vi "Ver 1.8.vi"() -> ()   [LabVIEW 2015]
uses:
  <instrlib>/Keithley 622x LV 2009/Configure/Source/Typedefs/KE622x -- Current Range.ctl
  <instrlib>/Keithley 622x LV 2009/Configure/Source/Typedefs/KE622x -- Current Ranges.ctl
  <instrlib>/Keithley 622x LV 2009/Typedefs/KE622x -- On Off Control.ctl
  <instrlib>/Keithley 622x LV 2009/Configure/Source/Typedefs/KE622x -- Voltage Limit.ctl
  <instrlib>/Keithley 622x LV 2009/Utility/Typedefs/KE622x -- Instrument Type.ctl
  <instrlib>/Keithley 2000/Public/Configure/Configure DC Volts.vi
  <userlib>/LV-Link3/PolySubVIs/DtCreateAinChan.vi
  <userlib>/LV-Link3/PolySubVIs/DtOLReadSingle.vi
  <instrlib>/Keithley 2000/Keithley 2000.lvlib
  <instrlib>/Keithley 622x LV 2009/Keithley 622x.lvlib
panel:
  out "MULTIPLE GRAPHS":cluster{dbl[], dbl[]}[](graph)
  in  "X-Axis":T1(ring)
  in  "Range":u8(ring)=20 items=["100nV", "200nV", "500nV", "1µV", "2µV", "5µV", "10µV", "20µV", "50µV", "100µV", "200µV", "500µV", "1mV", "2mV", "5mV", "10mV", "20mV", "50mV", "100mV", "200mV", "500mV", "1V"]
  in  "Display Type copy":u16(ring) items=["X %", "Y %", "X Calibrated", "Y Calibrated", "Mag %", "Mag Calibrated", "Phase Degrees", "Ratio", "ADC 1", "ADC 2", "ADC 3", "ADC 4 ", "Noise %", "Noise Calibrated", "Ref Frequency", "", ""]
  out "Units copy":string
  out "Display copy":dbl format="%.3f"
  out "Overload":bool
  out "Display":dbl format="%.3f"
  out "Units":string
  in  "Display Type":u16(ring) items=["X %", "Y %", "X Calibrated", "Y Calibrated", "Mag %", "Mag Calibrated", "Phase Degrees", "Ratio", "ADC 1", "ADC 2", "ADC 3", "ADC 4 ", "Noise %", "Noise Calibrated", "Ref Frequency", "", ""]
  in  "Time Constant":u16(ring) items=["MIN", "1ms", "3ms", "10ms", "30ms", "100ms", "300ms", "1s", "3s", "10s", "30s", "100s", "300s"]
  in  "Slope":u8(ring) items=["6db/octave", "12dB/octave"]
  in  "Dynamic Reserve":u16(ring) items=["High Stability", "Normal", "High Reserve"]
  in  "Auto Sensitivity":bool
  in  "Auto Measure":bool
  out "Task out":i32
  out "daq_error out":errorcluster
  out "6221_error_out":errorcluster
  out "2000_error_out":errorcluster
  out "5110_error_out":errorcluster
  out "Input Mode":i32(ring) items=[" Voltage Input (A or A-B) ", "Current Input 10E6 V/A", "Current Input 10E8 V/A"]
  out "5110":refnum<visa-resource-name>
  in  "GPIB Address":i8=12 min=1 max=32 step=1
  out "DAQ":dbl format="%#_13g"
  out "2000":dbl format="%#_13g"
  in  "Device":string(combo)
  in  "Channels":string="0"
  in  "Number \nof points":i32
  in  "Folder\nprename":string
  out "TIME GRAPH":cluster{dbl[], dbl[]}[](graph)
  out "T0":u32
  out "LIMIT":bool
  out "LIMIT":bool
  out "Error Code":string
  in  "Comments":string
  out "file":refnum<file>
  out "2000":refnum<visa-resource-name>
  out "6221":refnum<visa-resource-name>
  out "Step  (A)":dbl=5e-05 format="%#_3p"
  in  "Stop\ncurrent (A)":dbl=0.002 format="%#_6p"
  in  "Start \ncurrent (A)":dbl=0.001 format="%#_6p"
  in  "Check For SCPI Errors? (T)":bool=TRUE
  out "Interlock Tripped?":bool
  out "Compliance?":bool
  in  "Turn Off Output \nIf Compliance?":bool=TRUE
  in  "Turning ON/OFF\ncurrent output":T2=enum."On"
  in  "Range Selection":T3={"Auto Range?"=TRUE, "Man / Selected\nRange"=enum."2nA"}
  # "FILE CONFIGURATION"
  # "ADMIN PANEL"
  # "KEITHLEY 6221 CONFIGURATION (ADMIN ONLY)"
  # "KEITHLEY DAQ CONFIGURATION (ADMIN ONLY)"
  # "READINGS"
  # "PRINCETON LOCK-IN AMP (ADMIN ONLY)"
  # "I don't know what the hell it is,\njust don't touch it"
  # "SENSITIVITY"
  # "INPUT CONFIGURATION"
  # "START, STOP, STEP, CONFIGURATION"
  # "IF ON"
  # "Output Channels Time - Constant \nSlope & Dynamic Reserve"
  # "Compliance = Limiting output voltage\nThis switch determines if we want to switch \noff the current output if wee exceed compliance"
  # "LOCK-IN READINGS"
  # "RIGHT DISPLAY"
  # "LEFT DISPLAY"
  # "There is a safe switch at \nthe back of the instrument \nThis indicator shows if it is on"
  # "You have hit a damn jackpot \nby exceeding the limited voltage\nCongrats"
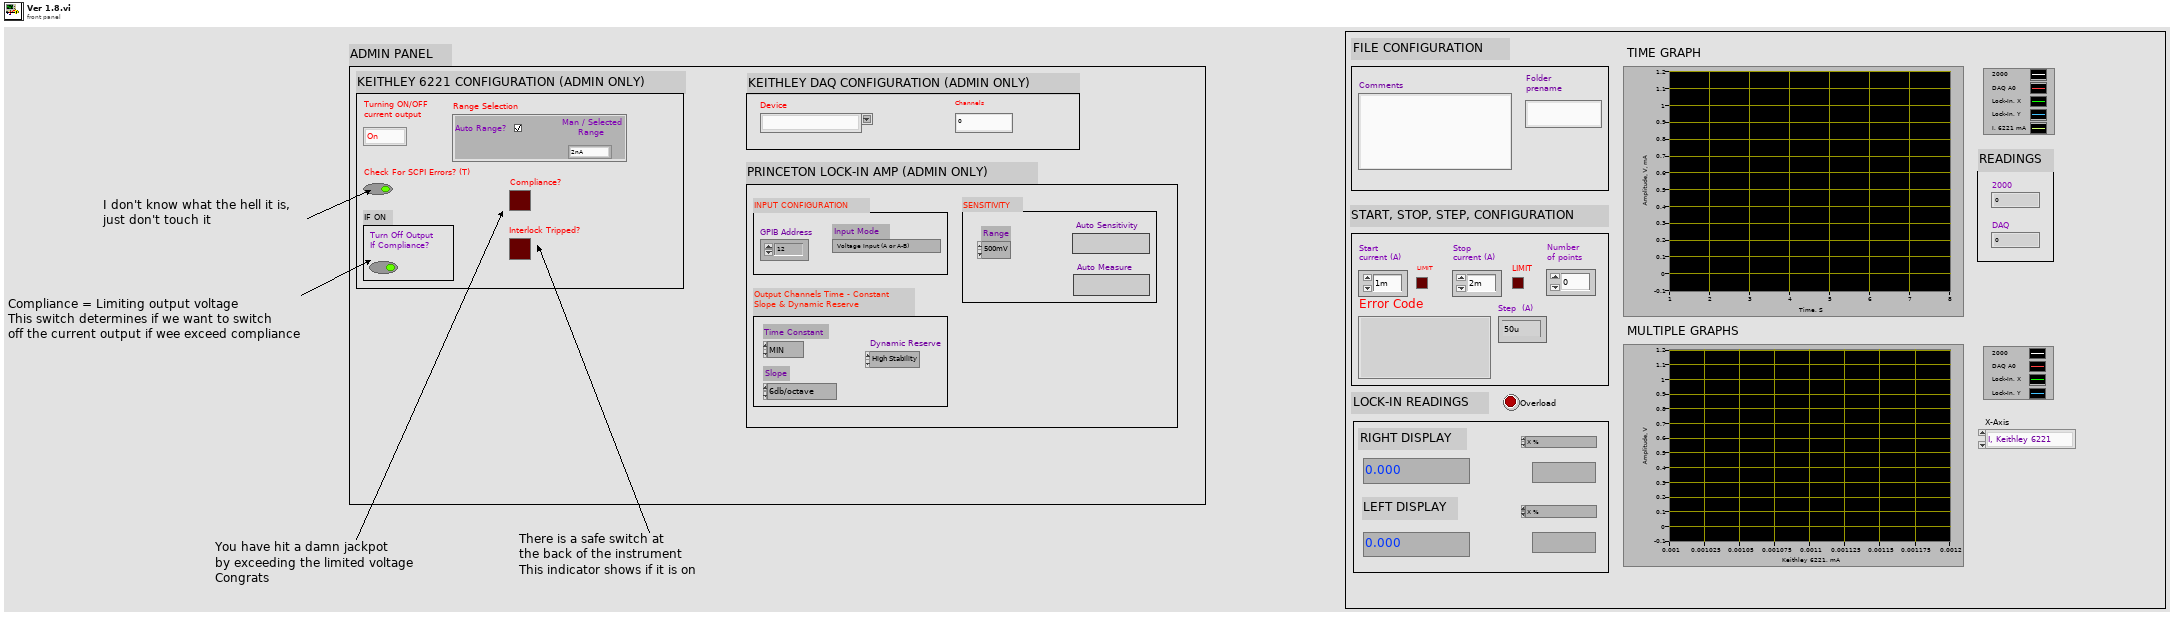
[diagram p1: front panel]
types:
  T1 = enum16{"I, Keithley 6221", "V, Keithley 2000", "V, Keithley DAQ", "V, Lock-In X", "V, Lock-In Y"}
  T2 = typedef "Keithley 622x.lvlib/KE622x -- On Off Control.ctl" = enum16{"Off", "On"}
  T3 = typedef "Keithley 622x.lvlib/KE622x -- Current Range.ctl" = cluster{"Auto Range?":bool, "Man / Selected\nRange":T4}
  T4 = typedef "Keithley 622x.lvlib/KE622x -- Current Ranges.ctl" = enum16{"2nA", "20nA", "200nA", "2uA", "20uA", "200uA", "2mA", "20mA", "100mA"}
  T5 = typedef "Keithley 622x.lvlib/KE622x -- Voltage Limit.ctl" = dbl
  T6 = typedef "Keithley 622x.lvlib/KE622x -- Instrument Type.ctl" = enum16{"KE6220", "KE6221"}
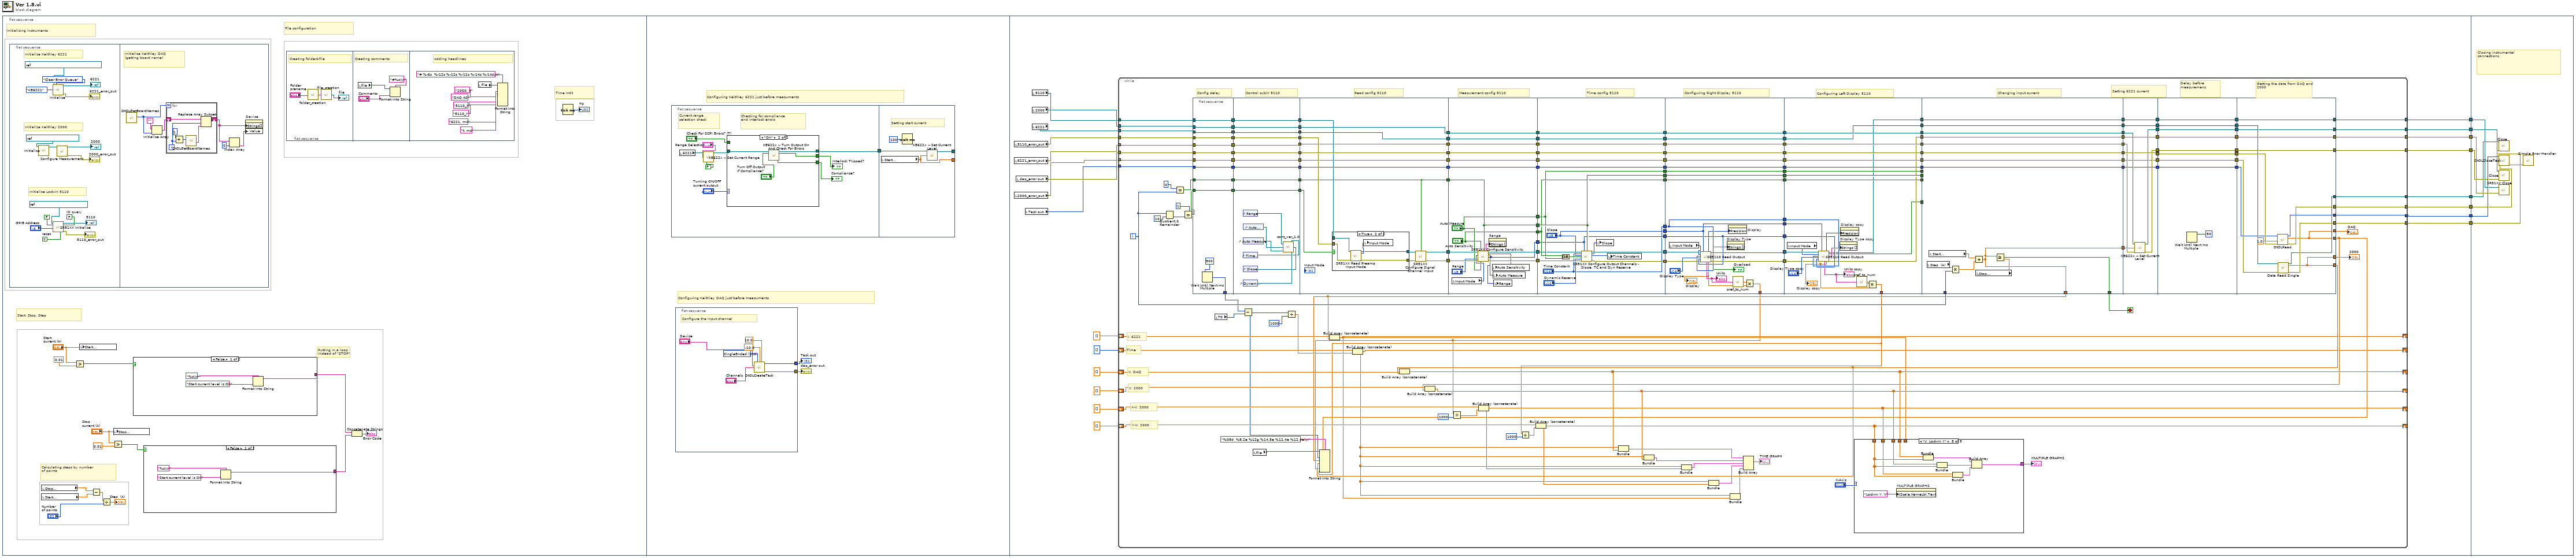
[diagram p0: block diagram]
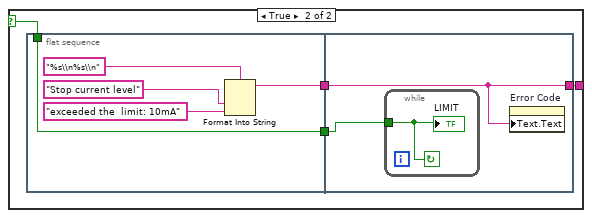
[diagram p2: hidden frame]
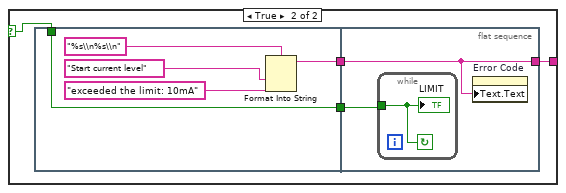
[diagram p3: hidden frame]
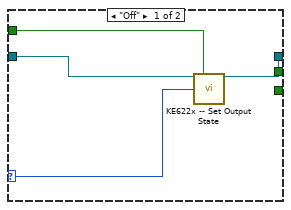
[diagram p4: hidden frame]
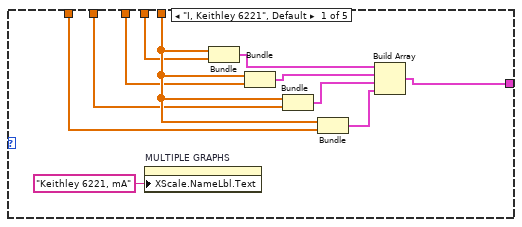
[diagram p5: hidden frame]
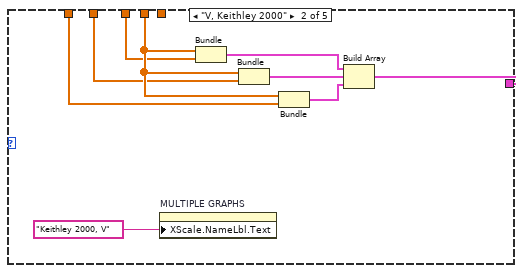
[diagram p6: hidden frame]
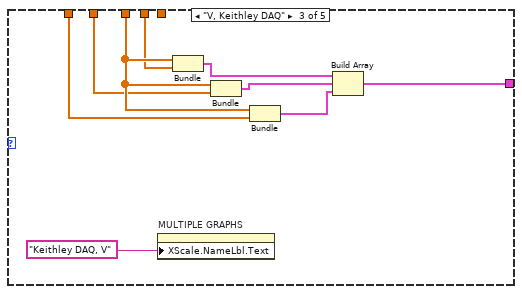
[diagram p7: hidden frame]
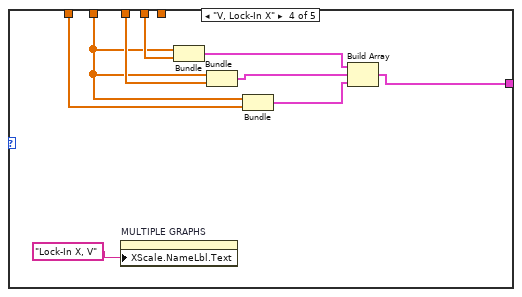
[diagram p8: hidden frame]
diagram:
  n1 = flat-sequence {
    tunnel: [w147] -> w8
    tunnel: [w145] -> w7
    tunnel: [w144] -> w6
    tunnel: [w143] -> w5
    tunnel: [w142] -> w4
    tunnel: [w141] -> w3
    tunnel: [w140] -> w2
    tunnel: [w139] -> w1
    tunnel: w8 -> [w560]
    tunnel: w7 -> [w559]
    tunnel: w6 -> [w558]
    tunnel: w5 -> [w557]
    tunnel: w4 -> [w556]
    tunnel: w3 -> [w555]
    tunnel: w2 -> [w554]
    tunnel: w1 -> [w553]
    frame #0 {
      # "Calculating steps by number\nof points"
      # "Time Intit"
      # "Putting in a loop \ninstead of \"STOP\""
      # "Start, Stop, Step"
      # "Initializing instruments"
      # "File configuration"
      n2 = flat-sequence {
        frame #0 {
          w31 = TRUE  # reset
          w30 = FALSE  # ID query
          # "Initialize Lock-In 5110"
          # "Initialize Keithley 2000"
          # "Initialize Keithley 6221"
          n3 = call <instrlib>:"Initialize.vi"("VISA resource name"=refnum<visa-resource-name> "KEITHLEY_MULTIMETER") -> ("VISA resource name out"=w35:refnum<visa-resource-name>)  [unwired: 17 in, 1 out]
          n4 = call <instrlib>:"Initialize.vi"("VISA resource name"=refnum<visa-resource-name> "KEITHLEY_DC_AC_CURRENT_SOURCE", "Error Queue Option"=enum16{"Clear Error Queue", "Error Query"}."Clear Error Queue", "Instrument Type"=KE622x_--_Instrument_Type."KE6221") -> ("VISA resource name out"=→"6221":refnum<visa-resource-name>, "error out"=→"6221_error_out":errorcluster)  [unwired: 11 in]
          n5 = call "SR51XX Initialize"("VISA session (for class)"=refnum<visa-resource-name> "LOCK_IN_5110_PRINCETON", "Interface"=FALSE, "ID query"=w30, "GPIB Address"="GPIB Address", "reset"=w31) -> ("VISA session"=→"5110":refnum<visa-resource-name>, "error out"=→"5110_error_out":errorcluster)  [unwired: 8 in, 1 out]
          n6 = call-poly <instrlib>:"Configure Measurement.vi"("VISA resource name"=w35) -> ("VISA resource name out"=→"2000":refnum<visa-resource-name>, "error out"=→"2000_error_out":errorcluster)  [unwired: 17 in]
        }
        frame #1 {
          # "Initialize Keithley DAQ \n(getting board name)"
          n7 = call <userlib>:"DtOLGetBoardNames.vi"() -> ("Number of boards"=w40:u32)  [unwired: 9 in, 2 out]
          n8 = Initialize Array("", w40) -> (w42:string[])
          n9 = for {
            N: w40 -> [_]
            shift-right: [w48] -> w45
            shift-left: w42 -> [w49]
            i -> [w47]
            n10 = Add(x=1, y=w47) -> (x+y=w51:i32)
            n11 = call <userlib>:"DtOLGetBoardNames.vi"("Select Board"=w51) -> ("Board Name"=w46:string)  [unwired: 8 in, 2 out]
            n12 = Replace Array Subset(array=w49, new element=w46, index=w47) -> (w48:string[])
          }
          n13 = Index Array(array=w45, index=0) -> (element=w44:string)
          n14 = property on="Device" class="CmbBox"("Strings[]"=w45, "Value"=w44) -> ()  [unwired: 2 in, 2 out]
        }
      }
      n15 = local read "Stop\ncurrent (A)"() -> (w12:dbl)
      n16 = local read "Start \ncurrent (A)"() -> (w11:dbl)
      n17 = Greater?(x="Start \ncurrent (A)", y=T5 0.01) -> (0:w19:bool)
      n18 = local write "Start \ncurrent (A)"("Start \ncurrent (A)") -> ()
      n19 = Subtract(x=w12, y=w11) -> (x-y=w9:dbl)
      n20 = Divide(x=w9, y="Number \nof points") -> (x/y=→"Step  (A)":dbl)
      n21 = Greater?(x="Stop\ncurrent (A)", y=T5 0.01) -> (0:w18:bool)
      n22 = local write "Stop\ncurrent (A)"("Stop\ncurrent (A)") -> ()
      n23 = case shown="False" w19 {
        selector: w19 -> [_ w71]
        tunnel: [w67 w73] -> w17
        frame False {
          n24 = Format Into String(format string="%s\\n", "Start current level is OK" ("false string")) -> (resulting string=w67:string)  [unwired: 2 in, 1 out]
        }
        frame True {
          n25 = flat-sequence {
            tunnel: [w75] -> w72
            tunnel: w71 -> [w74]
            tunnel: [w74] -> w70
            tunnel: [w79] -> w73
            tunnel: w72 -> [w79]
            tunnel: w70 -> [w80]
            frame #0 {
              n26 = Format Into String(format string="%s\\n%s\\n", "Start current level" ("String"), "exceeded the limit: 10mA" ("input 2")) -> (resulting string=w75:string)  [unwired: 2 in, 1 out]
            }
            frame #1 {
              n27 = while {
                tunnel: w80 -> [w81]
                stop <- w81 continue-if-true
                "LIMIT" <- w81
              }
              n28 = property on="Error Code" class="Str"("Text.Text"=w79) -> ()  [unwired: 2 in, 2 out]
            }
          }
        }
      }
      n29 = case shown="False" w18 {
        selector: w18 -> [_ w55]
        tunnel: [w52 w58] -> w16
        frame False {
          n30 = Format Into String(format string="%s\\n", "Start current level is OK" ("false string")) -> (resulting string=w52:string)  [unwired: 2 in, 1 out]
        }
        frame True {
          n31 = flat-sequence {
            tunnel: [w60] -> w57
            tunnel: [w59] -> w56
            tunnel: w55 -> [w59]
            tunnel: [w64] -> w58
            tunnel: w57 -> [w64]
            tunnel: w56 -> [w65]
            frame #0 {
              n32 = Format Into String(format string="%s\\n%s\\n", "Stop current level" ("String"), "exceeded the  limit: 10mA" ("input 2")) -> (resulting string=w60:string)  [unwired: 2 in, 1 out]
            }
            frame #1 {
              n33 = while {
                tunnel: w65 -> [w66]
                stop <- w66 continue-if-true
                "LIMIT" <- w66
              }
              n34 = property on="Error Code" class="Str"("Text.Text"=w64) -> ()  [unwired: 2 in, 2 out]
            }
          }
        }
      }
      n35 = flat-sequence {
        frame #0 {
          # "Creating folder&file"
          n36 = call "folder_creation.vi"("Name"="Folder\nprename") -> ("String"=w83:string)
          n37 = call "file_creation.vi"("String"=w83) -> ("refnum out"=→"file":refnum<file>)
        }
        frame #1 {
          # "Creating comments"
          n38 = local read "file"() -> (w85:refnum<file>)
          n39 = Format Into String(format string="#%s\\n", initial string=w85, "Comments") -> ()  [unwired: 1 in, 2 out]
        }
        frame #2 {
          # "Adding headlines"
          n40 = local read "file"() -> (w95:refnum<file>)
          n41 = Format Into String(format string="# %-6s  %-12s %-12s %-12s %-14s %-14s\\n", initial string=w95, "t, ms" ("input 3"), "6221, mA" ("input 3"), "2000, V" ("input 1"), "DAQ A0" ("input 2"), "5110_X" ("input 3"), "5110_Y " ("input 3")) -> ()  [unwired: 1 in, 2 out]
        }
      }
      n42 = Concatenate Strings(w17, w16) -> (→"Error Code":string)
      n43 = Tick Count (ms)() -> (millisecond timer value=→"T0":u32)
    }
    frame #1 {
      # "Configuring Keithley DAQ just before measuments"
      # "Configuring Keithley 6221 just before measuments"
      n44 = flat-sequence {
        tunnel: [w106] -> w98
        tunnel: [w124] -> _
        tunnel: [w126] -> _
        tunnel: w98 -> [w125]
        frame #0 {
          # "Current range \nselection check"
          # "Checking for compliance\nand interlock errors"
          n45 = local read "6221"() -> (w109:refnum<visa-resource-name>)
          n46 = call <instrlib>:"KE622x -- Set Current Range.vi"("Resource In"=w109, "Current Range In"="Range Selection", "Read Back Set Values? (T)"=FALSE) -> ("Resource Out (dupl)"=w114:refnum<visa-resource-name>)  [unwired: 10 in, 2 out]
          n47 = case shown="\"On\"" "Turning ON/OFF\ncurrent output" {
            selector: "Turning ON/OFF\ncurrent output" -> [w118 _]
            tunnel: [_ w122] -> w112
            tunnel: [_ w121] -> w113
            tunnel: "Check For SCPI Errors? (T)" -> [w117 _]
            tunnel: w114 -> [w115 w120]
            tunnel: [w116 w119] -> w106
            frame "Off" {
              n48 = call <instrlib>:"KE622x -- Set Output State.vi"("Resource In"=w115, "Check For SCPI Errors? (T)"=w117, "Output State"=w118) -> ("Resource Out (dupl)"=w116:refnum<visa-resource-name>)  [unwired: 11 in, 1 out]
            }
            frame "On" {
              n49 = call <instrlib>:"KE622x -- Turn Output On And Check For Errors.vi"("Resource In"=w120, "Turn Off Output If Compliance?"="Turn Off Output \nIf Compliance?") -> ("Resource Out (dupl)"=w119:refnum<visa-resource-name>, "Interlock Tripped?"=w122:bool, "Compliance?"=w121:bool)  [unwired: 10 in, 1 out]
            }
          }
          "Interlock Tripped?" <- w112
          "Compliance?" <- w113
        }
        frame #1 {
          # "Setting start current"
          n50 = local read "Start \ncurrent (A)"() -> (w124:dbl)
          n51 = Wait (ms)(milliseconds to wait=u32 100) -> ()  [unwired: 1 out]
          n52 = call <instrlib>:"KE622x -- Set Current Level.vi"("Resource In"=w125, "Current Level (A) In"=w124) -> ("Resource Out (dupl)"=w126:refnum<visa-resource-name>)  [unwired: 12 in, 1 out]
        }
      }
      n53 = flat-sequence {
        tunnel: [w100] -> w96
        tunnel: [w99] -> w97
        frame #0 {
          w104 = 100 items=["SingleEnded"=100, "Differential"=101] ("Channel Type")
          # "Configure the input channel"
          n54 = call-poly <userlib>:"DtOLCreateTask.vi"("Channel Type"=w104, "Range Min"=-10.0, "Range Max"=10.0, "Board Name"="Device", "Channel"="Channels") -> ("Task out"=w100:i32, "error out"=w99:errorcluster)  [unwired: 8 in, 1 out]
        }
      }
      "daq_error out" <- w97
      "Task out" <- w96
    }
    frame #2 {
      n55 = local read "5110_error_out"() -> (w132:errorcluster)
      n56 = local read "6221_error_out"() -> (w131:errorcluster)
      n57 = local read "2000_error_out"() -> (w129:errorcluster)
      n58 = local read "daq_error out"() -> (w130:errorcluster)
      n59 = local read "Task out"() -> (w128:i32)
      n60 = local read "5110"() -> (w135:refnum<visa-resource-name>)
      n61 = local read "2000"() -> (w134:refnum<visa-resource-name>)
      n62 = local read "6221"() -> (w133:refnum<visa-resource-name>)
      n63 = while {
        shift-right: [w200] -> _
        shift-left: dbl[] [] -> [w317]
        shift-right: [w152] -> _
        shift-left: i32[] [] -> [w316]
        tunnel: w134 -> [w314]
        tunnel: w133 -> [w313]
        tunnel: w130 -> [w301]
        tunnel: w128 -> [w297]
        tunnel: [w306] -> w147
        shift-right: [w199] -> _
        shift-left: dbl[] [] -> [w305]
        tunnel: [w293] -> w145
        tunnel: [w292] -> w144
        tunnel: [w291] -> w143
        tunnel: [w289] -> w142
        tunnel: [w286] -> w141
        tunnel: w135 -> [w282]
        tunnel: w132 -> [w281]
        tunnel: w131 -> [w273]
        tunnel: w129 -> [w272]
        tunnel: [w215] -> w140
        tunnel: [w212] -> w139
        shift-right: [w198] -> _
        shift-left: dbl[] [] -> [w211]
        shift-right: [w197] -> _
        shift-left: dbl[] [] -> [w210]
        shift-right: [w151] -> _
        shift-left: dbl[] [] -> [w201]
        i -> [w274]
        stop <- w307 stop-if-true
        # "Y-V, 2000"
        # "X-V, 2000"
        # "I, 6221"
        # "Config delay"
        # "Control subVI 5110"
        # "Read config 5110"
        # "Measurement config 5110"
        # "Time config 5110"
        # "Configuring Right Display 5110"
        # "Configuring Left Display 5110"
        # "Setting 6221 current"
        # "Delay before measuremens"
        # "Getting the data from DAQ and 2000"
        # "Changing input current"
        # "Time"
        # "V, DAQ"
        # "V, 2000"
        n64 = Quotient & Remainder(x=w274, y=10) -> (floor(x/y)=w279:i32)  [unwired: 1 out]
        n65 = Equal?(x=0, y=w274) -> (x = y?=w276:bool)
        n66 = Equal?(x=1, y=w279) -> (x = y?=w275:bool)
        n67 = flat-sequence {
          tunnel: w314 -> [w376]
          tunnel: [w376] -> w196
          tunnel: w313 -> [w375]
          tunnel: [w375] -> w194
          tunnel: [w373] -> w192
          tunnel: w301 -> [w373]
          tunnel: [w372] -> w190
          tunnel: w297 -> [w372]
          tunnel: w282 -> [w371]
          tunnel: [w371] -> w188
          tunnel: [w370] -> w186
          tunnel: w281 -> [w370]
          tunnel: w276 -> [w369]
          tunnel: [w369] -> w184
          tunnel: w275 -> [w368]
          tunnel: [w368] -> w182
          tunnel: w273 -> [w367]
          tunnel: [w367] -> w180
          tunnel: w272 -> [w366]
          tunnel: [w366] -> w178
          tunnel: [w365] -> w263
          tunnel: w196 -> [w392]
          tunnel: [w392] -> w195
          tunnel: w194 -> [w391]
          tunnel: [w391] -> w193
          tunnel: w192 -> [w390]
          tunnel: [w390] -> w191
          tunnel: w190 -> [w389]
          tunnel: [w389] -> w189
          tunnel: w188 -> [w388]
          tunnel: [w388] -> w187
          tunnel: w186 -> [w387]
          tunnel: [w387] -> w185
          tunnel: w184 -> [w386]
          tunnel: [w386] -> w183
          tunnel: w182 -> [w385]
          tunnel: [w385] -> w181
          tunnel: w180 -> [w384]
          tunnel: [w384] -> w179
          tunnel: w178 -> [w383]
          tunnel: [w383] -> w177
          tunnel: w195 -> [w406]
          tunnel: [w406] -> w262
          tunnel: w193 -> [w405]
          tunnel: [w405] -> w261
          tunnel: w191 -> [w404]
          tunnel: [w404] -> w260
          tunnel: w189 -> [w403]
          tunnel: [w403] -> w259
          tunnel: w187 -> [w402]
          tunnel: w185 -> [w399]
          tunnel: [w398] -> w258
          tunnel: [w397] -> w257
          tunnel: w183 -> [w396]
          tunnel: [w396] -> w256
          tunnel: w181 -> [w395]
          tunnel: w179 -> [w394]
          tunnel: [w394] -> w255
          tunnel: w177 -> [w393]
          tunnel: [w393] -> w254
          tunnel: w262 -> [w432]
          tunnel: [w432] -> w253
          tunnel: w261 -> [w431]
          tunnel: [w431] -> w252
          tunnel: w260 -> [w430]
          tunnel: [w430] -> w251
          tunnel: w259 -> [w429]
          tunnel: [w429] -> w250
          tunnel: w258 -> [w426]
          tunnel: [w425] -> w249
          tunnel: w257 -> [w424]
          tunnel: [w423] -> w248
          tunnel: w256 -> [w421]
          tunnel: [w421] -> w247
          tunnel: w255 -> [w428]
          tunnel: [w428] -> w246
          tunnel: w254 -> [w427]
          tunnel: [w427] -> w245
          tunnel: ["Auto Measure"] -> w244
          tunnel: ["Auto Sensitivity"] -> w243
          tunnel: [w416] -> w242
          tunnel: w253 -> [w452]
          tunnel: [w452] -> w176
          tunnel: w252 -> [w451]
          tunnel: [w451] -> w175
          tunnel: w251 -> [w450]
          tunnel: [w450] -> w174
          tunnel: w250 -> [w449]
          tunnel: [w449] -> w173
          tunnel: w249 -> [w442]
          tunnel: w248 -> [w440]
          tunnel: [w439] -> w172
          tunnel: w247 -> [w446]
          tunnel: [w446] -> w171
          tunnel: w246 -> [w448]
          tunnel: [w448] -> w170
          tunnel: w245 -> [w447]
          tunnel: [w447] -> w169
          tunnel: w244 -> [w444]
          tunnel: [w444] -> w168
          tunnel: w243 -> [w445]
          tunnel: [w445] -> w167
          tunnel: w242 -> [w435]
          tunnel: [w435] -> w166
          tunnel: [w441] -> w165
          tunnel: ["Time Constant"] -> w164
          tunnel: ["Slope"] -> w163
          tunnel: [w477] -> w241
          tunnel: [w476] -> w240
          tunnel: [w475] -> w239
          tunnel: [w474] -> w238
          tunnel: [w460] -> w237
          tunnel: [w473] -> w236
          tunnel: [w472] -> w235
          tunnel: [w471] -> w234
          tunnel: [w470] -> w233
          tunnel: [w469] -> w232
          tunnel: [w462] -> w231
          tunnel: [w465] -> w230
          tunnel: [w463] -> w229
          tunnel: [w468] -> w228
          tunnel: [w453] -> w150
          tunnel: w163 -> [w468]
          tunnel: w164 -> [w463]
          tunnel: w165 -> [w466]
          tunnel: w166 -> [w462]
          tunnel: w167 -> [w469]
          tunnel: w168 -> [w470]
          tunnel: w169 -> [w471]
          tunnel: w170 -> [w472]
          tunnel: w171 -> [w473]
          tunnel: w172 -> [w461]
          tunnel: w173 -> [w474]
          tunnel: w174 -> [w475]
          tunnel: w175 -> [w476]
          tunnel: w176 -> [w477]
          tunnel: w241 -> [w502]
          tunnel: [w502] -> w227
          tunnel: w240 -> [w501]
          tunnel: [w501] -> w226
          tunnel: w239 -> [w500]
          tunnel: [w500] -> w225
          tunnel: w238 -> [w499]
          tunnel: [w499] -> w224
          tunnel: w237 -> [w486]
          tunnel: w236 -> [w498]
          tunnel: [w498] -> w223
          tunnel: w235 -> [w497]
          tunnel: [w497] -> w222
          tunnel: w234 -> [w496]
          tunnel: [w496] -> w221
          tunnel: w233 -> [w495]
          tunnel: [w495] -> w220
          tunnel: w232 -> [w494]
          tunnel: [w494] -> w219
          tunnel: w231 -> [w487]
          tunnel: w230 -> [w484]
          tunnel: [w483] -> w218
          tunnel: w229 -> [w488]
          tunnel: w228 -> [w489]
          tunnel: [w485] -> w217
          tunnel: [w482] -> w216
          tunnel: [w478] -> w156
          tunnel: [w505] -> w311
          tunnel: w274 -> [w515]
          tunnel: [w511] -> w307
          tunnel: [w503] -> w309
          tunnel: [w513] -> w308
          tunnel: [w510] -> w302
          tunnel: [w509] -> w298
          tunnel: [w508] -> w271
          tunnel: [w507] -> w270
          tunnel: [w506] -> w269
          tunnel: [w504] -> w268
          tunnel: [w503] -> w159
          tunnel: w216 -> [_]
          tunnel: w217 -> [w506]
          tunnel: w218 -> [w504]
          tunnel: w219 -> [_]
          tunnel: w220 -> [_]
          tunnel: w221 -> [w508]
          tunnel: w222 -> [w507]
          tunnel: w223 -> [_]
          tunnel: w224 -> [w509]
          tunnel: w225 -> [w510]
          tunnel: w226 -> [w513]
          tunnel: w227 -> [w505]
          tunnel: w311 -> [w528]
          tunnel: [w528] -> w310
          tunnel: w309 -> [w527]
          tunnel: w308 -> [w526]
          tunnel: [w525] -> w303
          tunnel: w302 -> [w525]
          tunnel: [w524] -> w299
          tunnel: w298 -> [w524]
          tunnel: [w523] -> w290
          tunnel: [w522] -> w287
          tunnel: w271 -> [w520]
          tunnel: w270 -> [w521]
          tunnel: w269 -> [w518]
          tunnel: w268 -> [w519]
          tunnel: [w520] -> w267
          tunnel: [w519] -> w264
          tunnel: [w518] -> w213
          tunnel: w310 -> [w537]
          tunnel: [w537] -> w312
          tunnel: [w535] -> w304
          tunnel: w303 -> [w535]
          tunnel: [w534] -> w300
          tunnel: w299 -> [w534]
          tunnel: w290 -> [w533]
          tunnel: [w533] -> w288
          tunnel: w287 -> [w532]
          tunnel: [w532] -> w285
          tunnel: w267 -> [w531]
          tunnel: [w531] -> w266
          tunnel: [w530] -> w265
          tunnel: w264 -> [w530]
          tunnel: [w529] -> w214
          tunnel: w213 -> [w529]
          tunnel: w312 -> [w552]
          tunnel: [w541] -> w157
          tunnel: [w550] -> w306
          tunnel: w304 -> [w549]
          tunnel: w300 -> [w548]
          tunnel: [w542] -> w154
          tunnel: [w547] -> w293
          tunnel: [w546] -> w292
          tunnel: [w545] -> w291
          tunnel: [w544] -> w289
          tunnel: w288 -> [w544]
          tunnel: [w543] -> w286
          tunnel: w285 -> [w543]
          tunnel: [w542] -> w284
          tunnel: [w541] -> w283
          tunnel: w266 -> [w540]
          tunnel: w265 -> [w539]
          tunnel: [w539] -> w215
          tunnel: w214 -> [w538]
          tunnel: [w538] -> w212
          frame #0 {
            n68 = Wait Until Next ms Multiple(millisecond multiple=u32 500) -> (millisecond timer value=w365:u32)
          }
          frame #1 {
            n69 = control-ref of="Range"() -> (w382:refnum<vi>)
            n70 = control-ref of="Auto Sensitivity"() -> (w381:refnum<vi>)
            n71 = control-ref of="Auto Measure"() -> (w380:refnum<vi>)
            n72 = control-ref of="Time Constant"() -> (w377:refnum<vi>)
            n73 = control-ref of="Slope"() -> (w378:refnum<vi>)
            n74 = control-ref of="Dynamic Reserve"() -> (w379:refnum<vi>)
            n75 = call "cont_ver_1.0.vi"("Dynamic Reserve"=w379, "Slope"=w378, "Time Constant"=w377, "Auto Measure"=w380, "Auto Sensitivity"=w381, "Range"=w382) -> ()
          }
          frame #2 {
            n76 = case shown="True" w395 {
              tunnel: w402 -> [w408 w413]
              tunnel: [w407 w411] -> w401
              tunnel: [w408 w410] -> w400
              tunnel: w399 -> [w407 w409]
              frame False {
              }
              frame True {
                n77 = call "SR51XX Read Preamp Input Mode"("VISA session (for class)"=w413, "error in (no error)"=w409) -> ("VISA session"=w410:refnum<visa-resource-name>, "Input Mode"=w412:i32, "error out"=w411:errorcluster)  [unwired: 15 in]
                n78 = local write "Input Mode"(w412) -> ()
              }
            }
            n79 = call "SR51XX Configure Signal Channel Input"("VISA session (for class)"=w400, "error in (no error)"=w401, "Update"=w396) -> ("VISA session"=w398:refnum<visa-resource-name>, "error out"=w397:errorcluster)  [unwired: 15 in]
          }
          frame #3 {
            n80 = local read "Input Mode"() -> (w422:i32)
            n81 = call "SR51XX Configure Sensitivity"("VISA session (for class)"=w426, "Input Mode"=w422, "Range"="Range", "error in (no error)"=w424, "Auto Sensitivity"="Auto Sensitivity", "Auto Measure"="Auto Measure", "Update"=w421) -> ("Range Annotations Out[]"=w414:string[], "VISA session"=w425:refnum<visa-resource-name>, "Auto Sensitivity out"=w418:bool, "Auto Measure out"=w417:bool, "Range Out"=w416:u8, "error out"=w423:errorcluster)  [unwired: 7 in]
            n82 = property on="Range" class="Ring (strict)"("Strings []"=w414) -> ()  [unwired: 2 in, 2 out]
            n83 = local write "Auto Sensitivity"(w418) -> ()
            n84 = local write "Auto Measure"(w417) -> ()
            n85 = local write "Range"(w416) -> ()
          }
          frame #4 {
            n86 = Or(x=w445, y=w444) -> (x .or. y?=w443:bool)
            n87 = call "SR51XX Configure Output Channels - Slope, TC and Dyn Reserve"("VISA session (for class)"=w442, "Time Constant"="Time Constant", "Slope"="Slope", "Check TC"=w443, "Dynamic Reserve"="Dynamic Reserve", "error in (no error)"=w440, "Range"=w435, "Update"=w446) -> ("VISA session"=w441:refnum<visa-resource-name>, "Slope Out"=w436:u8, "Time Constant Out"=w437:u16, "error out"=w439:errorcluster)  [unwired: 8 in]
            n88 = local write "Slope"(w436) -> ()
            n89 = local write "Time Constant"(w437) -> ()
          }
          frame #5 {
            n90 = local read "Input Mode"() -> (w467:i32)
            n91 = call "SR5110 Read Output"("VISA session (for class)"=w466, "Input Mode"=w467, "Time Constant"=w463, "Display Type"="Display Type", "Range"=w462, "error in (no error)"=w461, "Slope"=w468) -> ("Units"=w455:string, "Display Precision"=w459:i32, "Display"=w454:dbl, "VISA session"=w465:refnum<visa-resource-name>, "Available Display Types Out"=w458:string[], "Overload"=→"Overload":bool, "error out"=w460:errorcluster)  [unwired: 4 in, 2 out]
            "Units" <- w455
            "Display" <- w454
            n92 = property on="Display Type" class="Ring (strict)"("Strings []"=w458) -> ()  [unwired: 2 in, 2 out]
            n93 = property on="Display" class="DigNum (strict)"("Precision"=w459) -> ()  [unwired: 2 in, 2 out]
            n94 = call "pref_to_num.vi"("string"=w455) -> ("Numeric"=w456:dbl)
            n95 = Multiply(x=w456, y=w454) -> (x*y=w453:dbl)
          }
          frame #6 {
            n96 = local read "Input Mode"() -> (w493:i32)
            n97 = call "SR5110 Read Output"("VISA session (for class)"=w484, "Input Mode"=w493, "Time Constant"=w488, "Display Type"="Display Type copy", "Range"=w487, "error in (no error)"=w486, "Slope"=w489) -> ("Units"=w481:string, "Display Precision"=w490:i32, "Display"=w480:dbl, "VISA session"=w483:refnum<visa-resource-name>, "Reference Unlock"=w482:bool, "Available Display Types Out"=w491:string[], "error out"=w485:errorcluster)  [unwired: 4 in, 2 out]
            "Display copy" <- w480
            "Units copy" <- w481
            n98 = property on="Display Type copy" class="Ring (strict)"("Strings []"=w491) -> ()  [unwired: 2 in, 2 out]
            n99 = property on="Display copy" class="DigNum (strict)"("Precision"=w490) -> ()  [unwired: 2 in, 2 out]
            n100 = call "pref_to_num.vi"("string"=w481) -> ("Numeric"=w479:dbl)
            n101 = Multiply(x=w479, y=w480) -> (x*y=w478:dbl)
          }
          frame #7 {
            n102 = local read "Step  (A)"() -> (w516:dbl)
            n103 = local read "Start \ncurrent (A)"() -> (w517:dbl)
            n104 = Multiply(x=w516, y=w515) -> (x*y=w514:dbl)
            n105 = Add(x=w517, y=w514) -> (x+y=w503:dbl)
            n106 = local read "Stop\ncurrent (A)"() -> (w512:dbl)
            n107 = Greater Or Equal?(x=w503, y=w512) -> (x >= y?=w511:bool)
          }
          frame #8 {
            n108 = call <instrlib>:"KE622x -- Set Current Level.vi"("Resource In"=w526, "Current Level (A) In"=w527, "error in (no error)"=w521) -> ("Resource Out (dupl)"=w522:refnum<visa-resource-name>, "error out"=w523:errorcluster)  [unwired: 11 in]
          }
          frame #9 {
            n109 = Wait Until Next ms Multiple(millisecond multiple=u32 50) -> ()  [unwired: 1 out]
          }
          frame #10 {
            n110 = call-poly <userlib>:"DtOLRead.vi"("error in (no error)"=w549, "Timeout"=1.0, "Task in"=w548) -> ("error out"=w545:errorcluster, "Data Out"=w542:dbl, "Task out"=w550:i32)  [unwired: 6 in]
            n111 = call <instrlib>:"Data Read Single.vi"("VISA resource name"=w552, "error in (no error)"=w540) -> ("VISA resource name out"=w546:refnum<visa-resource-name>, "Measurement"=w541:dbl, "error out"=w547:errorcluster)  [unwired: 13 in, 2 out]
          }
        }
        n112 = local read "T0"() -> (w315:u32)
        n113 = Subtract(x=w263, y=w315) -> (x-y=w158:u32)
        n114 = local read "file"() -> (w162:refnum<file>)
        n115 = Divide(x=w158, y=u32 1000) -> (x/y=w160:dbl)
        n116 = Format Into String(format string="%08d  %8.2e %12g %14.5e %12.4e %12.4e\\n", initial string=w162, w158, w159, w157, w154, w150, w156) -> ()  [unwired: 1 in, 2 out]
        n117 = Build Array (concatenate)(w201, w159) -> (w151:dbl[])
        n118 = Build Array (concatenate)(w316, w160) -> (w152:dbl[])
        n119 = Build Array (concatenate)(w317, w157) -> (w200:dbl[])
        n120 = Build Array (concatenate)(w305, w154) -> (w199:dbl[])
        n121 = Divide(x=w150, y=u32 1000) -> (x/y=w205:dbl)
        n122 = Build Array (concatenate)(w211, w205) -> (w198:dbl[])
        n123 = Divide(x=w156, y=u32 1000) -> (x/y=w203:dbl)
        n124 = Build Array (concatenate)(w210, w203) -> (w197:dbl[])
        n125 = Bundle(w152, w200) -> (w295:cluster{dbl[], dbl[]})  [unwired: 1 in]
        n126 = Bundle(w152, w199) -> (w294:cluster{dbl[], dbl[]})  [unwired: 1 in]
        n127 = Bundle(w152, w198) -> (w209:cluster{dbl[], dbl[]})  [unwired: 1 in]
        n128 = Bundle(w152, w197) -> (w208:cluster{dbl[], dbl[]})  [unwired: 1 in]
        n129 = Bundle(w152, w151) -> (w153:cluster{dbl[], dbl[]})  [unwired: 1 in]
        n130 = Build Array(w295, w294, w209, w208, w153) -> (→"TIME GRAPH":cluster{dbl[], dbl[]}[])
        n131 = case shown="\"V, Lock-In Y\"" "X-Axis" {
          tunnel: w151 -> [w324 _ _ _ _]
          tunnel: w200 -> [w323 w337 w345 w352 w363]
          tunnel: w199 -> [w322 w333 w346 w351 w362]
          tunnel: w198 -> [w321 w332 w344 w350 w361]
          tunnel: w197 -> [w320 w331 w343 w349 w364]
          tunnel: [w319 w330 w339 w348 w357] -> w155
          frame "I, Keithley 6221", Default {
            n132 = property on="MULTIPLE GRAPHS" class="XYGraph (strict)"("XScale.NameLbl.Text"="Keithley 6221, mA" ("X Scale.Name Label.Text")) -> ()  [unwired: 2 in, 2 out]
            n133 = Bundle(w324, w323) -> (w325:cluster{dbl[], dbl[]})  [unwired: 1 in]
            n134 = Bundle(w324, w322) -> (w326:cluster{dbl[], dbl[]})  [unwired: 1 in]
            n135 = Bundle(w324, w321) -> (w327:cluster{dbl[], dbl[]})  [unwired: 1 in]
            n136 = Bundle(w324, w320) -> (w328:cluster{dbl[], dbl[]})  [unwired: 1 in]
            n137 = Build Array(w325, w326, w327, w328) -> (w319:cluster{dbl[], dbl[]}[])
          }
          frame "V, Keithley 2000" {
            n138 = property on="MULTIPLE GRAPHS" class="XYGraph (strict)"("XScale.NameLbl.Text"="Keithley 2000, V" ("X Scale.Name Label.Text")) -> ()  [unwired: 2 in, 2 out]
            n139 = Bundle(w337, w333) -> (w336:cluster{dbl[], dbl[]})  [unwired: 1 in]
            n140 = Bundle(w337, w332) -> (w335:cluster{dbl[], dbl[]})  [unwired: 1 in]
            n141 = Bundle(w337, w331) -> (w334:cluster{dbl[], dbl[]})  [unwired: 1 in]
            n142 = Build Array(w336, w335, w334) -> (w330:cluster{dbl[], dbl[]}[])
          }
          frame "V, Keithley DAQ" {
            n143 = property on="MULTIPLE GRAPHS" class="XYGraph (strict)"("XScale.NameLbl.Text"="Keithley DAQ, V" ("X Scale.Name Label.Text")) -> ()  [unwired: 2 in, 2 out]
            n144 = Bundle(w346, w345) -> (w340:cluster{dbl[], dbl[]})  [unwired: 1 in]
            n145 = Bundle(w346, w344) -> (w341:cluster{dbl[], dbl[]})  [unwired: 1 in]
            n146 = Bundle(w346, w343) -> (w342:cluster{dbl[], dbl[]})  [unwired: 1 in]
            n147 = Build Array(w340, w341, w342) -> (w339:cluster{dbl[], dbl[]}[])
          }
          frame "V, Lock-In X" {
            n148 = property on="MULTIPLE GRAPHS" class="XYGraph (strict)"("XScale.NameLbl.Text"="Lock-In X, V" ("X Scale.Name Label.Text")) -> ()  [unwired: 2 in, 2 out]
            n149 = Bundle(w350, w352) -> (w353:cluster{dbl[], dbl[]})  [unwired: 1 in]
            n150 = Bundle(w350, w351) -> (w354:cluster{dbl[], dbl[]})  [unwired: 1 in]
            n151 = Bundle(w350, w349) -> (w355:cluster{dbl[], dbl[]})  [unwired: 1 in]
            n152 = Build Array(w353, w354, w355) -> (w348:cluster{dbl[], dbl[]}[])
          }
          frame "V, Lock-In Y" {
            n153 = property on="MULTIPLE GRAPHS" class="XYGraph (strict)"("XScale.NameLbl.Text"="Lock-In Y, V" ("X Scale.Name Label.Text")) -> ()  [unwired: 2 in, 2 out]
            n154 = Bundle(w363, w364) -> (w360:cluster{dbl[], dbl[]})  [unwired: 1 in]
            n155 = Bundle(w362, w364) -> (w359:cluster{dbl[], dbl[]})  [unwired: 1 in]
            n156 = Bundle(w361, w364) -> (w358:cluster{dbl[], dbl[]})  [unwired: 1 in]
            n157 = Build Array(w360, w359, w358) -> (w357:cluster{dbl[], dbl[]}[])
          }
        }
        "MULTIPLE GRAPHS" <- w155
        "2000" <- w283
        "DAQ" <- w284
      }
    }
    frame #3 {
      # "Closing instrumental \nconnections"
      n158 = call <instrlib>:"Close.vi"("VISA resource name"=w558, "error in (no error)"=w559) -> ()  [unwired: 17 in, 1 out]
      n159 = call <userlib>:"DtOLCloseTask.vi"("Error in"=w557, "Task in"=w560) -> ("Error Out"=w561:errorcluster)  [unwired: 9 in]
      n160 = call <instrlib>:"Close.vi"("VISA resource name"=w555, "error in (no error)"=w556) -> ()  [unwired: 13 in, 1 out]
      n161 = call "SR51XX Close"("error in (no error)"=w553, "VISA session"=w554) -> ()  [unwired: 1 out]
      n162 = call <vilib>:"Simple Error Handler.vi"("error in (no error)"=w561) -> ()  [unwired: 4 in, 5 out]
    }
  }
